vi "Poll Sample Line Valve Control.vi"(8 "error in (no error)":errorcluster, 11 "Sample Line in":refnum<class "Sample Line.lvclass">) -> ()   [LabVIEW 2015, in "cRIO-Carbondioxide.lvlib" / "CO2-Actor.lvlib" / "Sample Line.lvclass"]
uses:
  Sample Line.lvclass
  Sample Line.lvclass/Sample Line.ctl
  Controls/Sample Line State Enumerator.ctl
  <vilib>/ActorFramework/Actor/Actor.lvclass/Actor.ctl
  <vilib>/ActorFramework/Message Enqueuer/Message Enqueuer.lvclass/Message Enqueuer.ctl
  Sample Line Messages/Open Line Msg/Open Line Msg.lvclass/Open Line Msg.ctl
  <vilib>/ActorFramework/Actor/Read Self Enqueuer.vi
  <vilib>/ActorFramework/Message Enqueuer/Enqueue.vi
  <vilib>/ActorFramework/Message Enqueuer/Init from Existing Queue.vi
  <vilib>/ActorFramework/Message Priority Queue/Priority Enqueue.vi
  <vilib>/ActorFramework/Actor/Actor.lvclass
  <vilib>/ActorFramework/Message Enqueuer/Message Enqueuer.lvclass
  Sample Line Messages/Open Line Msg/Open Line Msg.lvclass
  CO2 Actor/CO2 Actor.lvclass
  cRIO-CO2/cRIO-CO2.lvclass
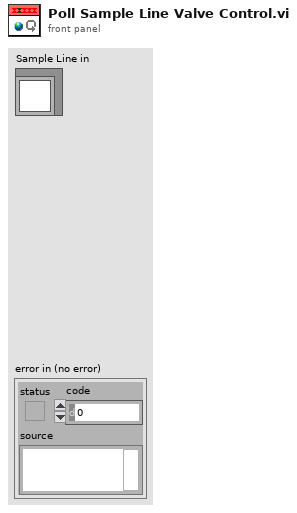
[diagram p1: front panel]
types:
  T1 = typedef "Sample Line State Enumerator.ctl" = enum16{"All lines closed", "Sample line 1.", "Sample line 2.", "Sample line 3.", "Sample line 4.", "Sample line 5.", "Out of range"}
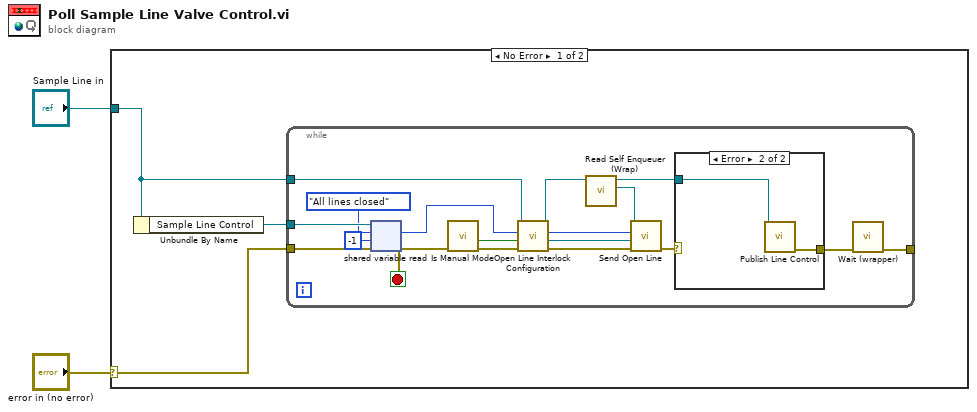
[diagram p0: block diagram]
diagram:
  n1 = case shown="No Error" "error in (no error)" {
    selector: "error in (no error)" -> [w3 _]
    tunnel: "Sample Line in" -> [w4 _]
    frame No Error {
      n2 = Unbundle By Name(w4) -> ("Sample Line Control"=w5:refnum<k21>)
      n3 = while {
        tunnel: w3 -> [w22]
        tunnel: w5 -> [w21]
        tunnel: w4 -> [w18]
        tunnel: [w6] -> _
        stop <- w11 stop-if-true
        n4 = shared-variable-read(w21, w22, -1 ("timeout ms"), Sample_Line_State_Enumerator."All lines closed" ("Enum")) -> (w11:errorcluster, w9:T1)  [unwired: 3 out]
        n5 = call "Is Manual Mode.vi"("error in (no error)"=w11) -> ("error out"=w10:errorcluster, "Manual Mode?"=w8:bool)  [unwired: 9 in]
        n6 = call "Open Line Interlock Configuration.vi"("error in (no error)"=w10, "Manual Mode (False)"=w8, "Sample Line (All Closed)"=w9, "Sample Line in"=w18) -> ("error out"=w20:errorcluster, "Interlock Chain"=w19:refnum<class "Interlock Chain.lvclass">, 2:"Sample Line out"=w16:T1, 3:"Sample Line out"=w17:refnum<class "Sample Line.lvclass">)  [unwired: 4 in]
        n7 = call "Read Self Enqueuer (Wrap).vi"("CO2 Actor in"=w17) -> ("Actor Framework:Message Enqueuer"=w15:refnum<class "Message Enqueuer.lvclass">, "CO2 Actor out"=w12:refnum<class "Sample Line.lvclass">)  [unwired: 9 in]
        n8 = call "Send Open Line.vi"("error in (no error)"=w20, "Interlock Chain"=w19, "Sample Line (All Closed)"=w16, "Message Enqueuer"=w15) -> ("error out"=w13:errorcluster)  [unwired: 6 in, 1 out]
        n9 = case shown="Error" w13 {
          tunnel: w12 -> [_ w24]
          tunnel: [_ w25] -> w7
          frame No Error {
          }
          frame Error {
            n10 = call "Publish Line Control.vi"("Sample Line in"=w24) -> ("error out"=w25:errorcluster)  [unwired: 9 in, 1 out]
          }
        }
        n11 = call "Wait (wrapper).vi"("error in (no error)"=w7) -> ("error out"=w6:errorcluster)  [unwired: 10 in]
      }
    }
    frame Error {
    }
  }
